vi "replaceFieldTokens.vi"(8 "error in (no error)":errorcluster, 10 "Query In":string, 11 "CreditTransaction in":refnum<class "CreditTransaction.lvclass">) -> (0 "error out":errorcluster, 2 "Query Out":string, 3 "CreditTransaction out":refnum<class "CreditTransaction.lvclass">)   [LabVIEW 2018, in "CreditTransaction.lvclass"]
uses:
  CreditTransaction.lvclass
  Transaction/Transaction.lvclass
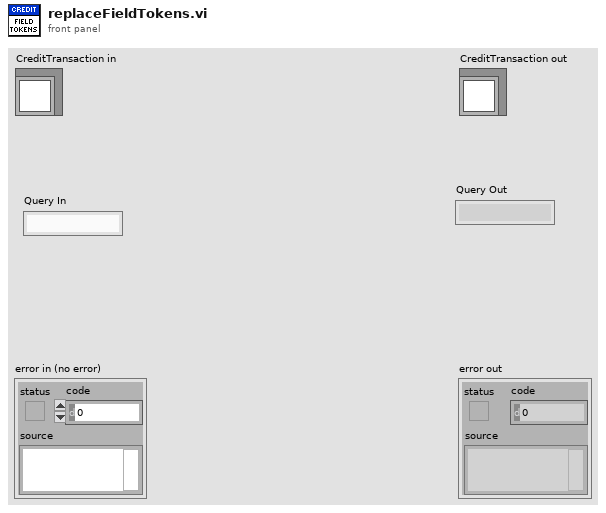
[diagram p1: front panel]
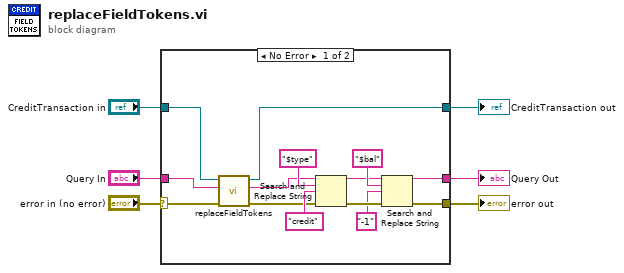
[diagram p0: block diagram]
diagram:
  n1 = case shown="No Error" "error in (no error)" {
    selector: "error in (no error)" -> [w8 w22]
    tunnel: [w20 w23] -> w1
    tunnel: "Query In" -> [w19 w21]
    tunnel: "CreditTransaction in" -> [w13 w23]
    tunnel: [w10 w22] -> w5
    tunnel: [w9 w21] -> w4
    frame No Error {
      n2 = call-parent "replaceFieldTokens.vi"("error in (no error)"=w8, "Query In"=w19, "Transaction in"=w13) -> ("error out"=w15:errorcluster, "Query Out"=w16:string, "Transaction out"=w20:refnum<class "CreditTransaction.lvclass">)  [unwired: 6 in]
      n3 = Search and Replace String(input string=w16, search string="$type", replace string="credit" ("replace string (\"\")"), error in=w15) -> (result string=w12:string, error out=w11:errorcluster)  [unwired: 4 in, 2 out]
      n4 = Search and Replace String(input string=w12, search string="$bal", replace string="-1" ("replace string (\"\")"), error in=w11) -> (result string=w9:string, error out=w10:errorcluster)  [unwired: 4 in, 2 out]
    }
    frame Error {
    }
  }
  "error out" <- w5
  "CreditTransaction out" <- w1
  "Query Out" <- w4
